vi "DllSqrtTemp.vi"(8 "ready for output":bool, 9 "input valid":bool, 11 "radicand":fxp<+/-,64,32>) -> (0 "ready for input":bool, 1 "output valid":bool, 2 "ovfl?":bool, 3 "sqrt":fxp<+/-,64,32>)   [LabVIEW 2017]
uses:
  <vilib>/rvi/FXPMathLib/FxpSqrt/subVIs/nifxpmath_Sqrt_SimConfig.ctl
  <vilib>/fxp/LVFixedPointOverflowPolicyTypeDef.ctl
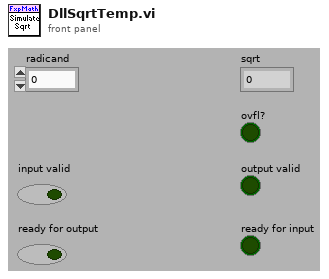
[diagram p1: front panel]
types:
  T1 = typedef "nifxpmath_Sqrt_SimConfig.ctl" = cluster{"kRadicandLen":u16, "kRadicandIwl":i16, "kSqrtLen":u16, "kRoundup":bool, "overflow mode":T2, "kCycleLimit":u16, "kStrictLimit":bool, "kSupportSCTL":bool, "kOutputReg":bool, "kInputReg":bool}
  T2 = typedef "LVFixedPointOverflowPolicyTypeDef.ctl" = enum32{"Wrap", "Saturate"}
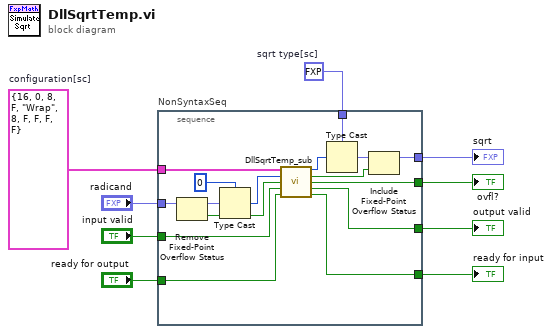
[diagram p0: block diagram]
diagram:
  w1 = T1 {"kRadicandLen"=16, "kRadicandIwl"=0, "kSqrtLen"=8, "kRoundup"=FALSE, "overflow mode"=enum."Wrap", "kCycleLimit"=8, "kStrictLimit"=FALSE, "kSupportSCTL"=FALSE, "kOutputReg"=FALSE, "kInputReg"=FALSE}  # configuration[sc]
  w4 = fxp<+/-,64,32> 0.0  # sqrt type[sc]
  n1 = stacked-sequence "NonSyntaxSeq" {
    tunnel: "input valid" -> [w18]
    tunnel: [w11] -> w8
    tunnel: [w10] -> w7
    tunnel: [w12] -> w6
    tunnel: [w15] -> w3
    tunnel: w1 -> [w21]
    tunnel: "radicand" -> [w23]
    tunnel: w4 -> [w24]
    tunnel: "ready for output" -> [w17]
    frame #0 {
      n2 = Remove Fixed-Point Overflow Status(3:w23) -> (0:w19:bool, 1:w22:fxp<+/-,64,32>)
      n3 = Type Cast(type=u64 0, x=w22) -> (*(type *) &x=w20:u64)
      n4 = call <vilib>:"DllSqrtTemp_sub.vi"("configuration[sc]"=w21, "x"=w20, "x ovfl status"=w19, "input valid"=w18, "ready for output"=w17) -> ("sqrt"=w13:u64, "sqrt ovfl status"=w14:bool, "operational overflow"=w12:bool, "output valid"=w11:bool, "ready for input"=w10:bool)  [unwired: 6 out]
      n5 = Type Cast(type=w24, x=w13) -> (*(type *) &x=w16:fxp<+/-,64,32>)
      n6 = Include Fixed-Point Overflow Status(2:w14, 3:w16) -> (1:w15:fxp<+/-,64,32>)
    }
  }
  "output valid" <- w8
  "ready for input" <- w7
  "ovfl?" <- w6
  "sqrt" <- w3
